vi "Configure Network De-embedding.vi"(0 "VISA resource name":refnum<visa-resource-name>, 1 "Channel (1)":i32=1, 2 "Network De-embeding State (F: Disable)":bool, 3 "Port 1 (1)":i32=1, 5 "Circuit Type (0: None)":u16(ring) items=["None", "User"], 11 "error in (no error)":errorcluster, 14 "File Name (\"\")":string) -> (4 "VISA resource name out":refnum<visa-resource-name>, 15 "error out":errorcluster)   [LabVIEW 2022 SP3, in "Agilent ENA Series.lvlib"]
doc: "Configures network de-embedding."
uses:
  <instrlib>/Agilent ENA Series/Agilent ENA Series.lvlib
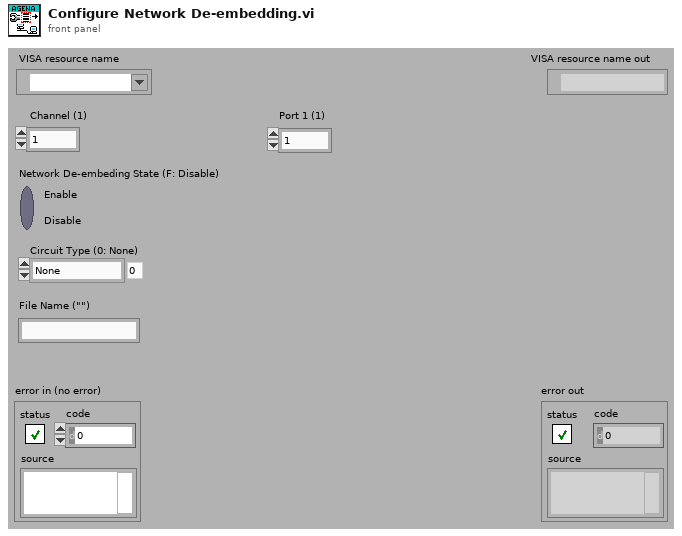
[diagram p1: front panel]
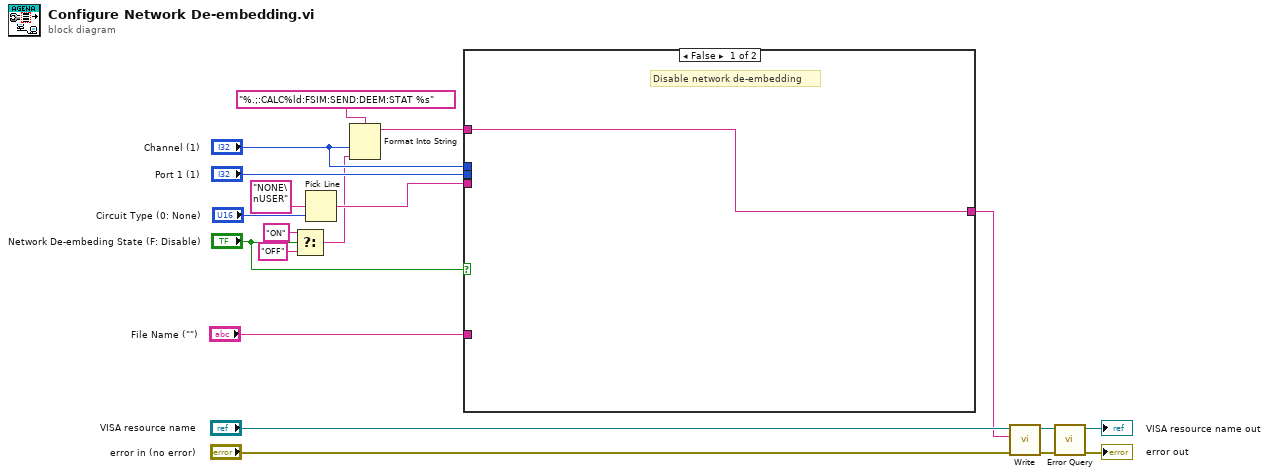
[diagram p0: block diagram]
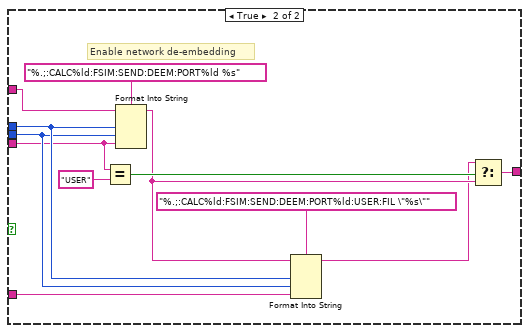
[diagram p2: hidden frame]
diagram:
  n1 = Select(t="ON", s="Network De-embeding State (F: Disable)", f="OFF") -> (s? t:f=w7:string)
  n2 = Pick Line(multi-line string="NONE\nUSER", line index="Circuit Type (0: None)") -> (output string=w12:string)  [unwired: 1 in]
  n3 = Format Into String(format string="%.;:CALC%ld:FSIM:SEND:DEEM:STAT %s", "Channel (1)", w7) -> (resulting string=w5:string)  [unwired: 2 in, 1 out]
  n4 = case shown="False" "Network De-embeding State (F: Disable)" {
    tunnel: "Channel (1)" -> [_ w28]
    tunnel: "Port 1 (1)" -> [_ w27]
    tunnel: w12 -> [_ w26]
    tunnel: "File Name (\"\")" -> [_ w21]
    tunnel: [w20 w23] -> w6
    tunnel: w5 -> [w20 w22]
    frame False {
      # "Disable network de-embedding"
    }
    frame True {
      # "Enable network de-embedding"
      n5 = Equal?(x=w26, y="USER") -> (x = y?=w30:bool)
      n6 = Format Into String(format string="%.;:CALC%ld:FSIM:SEND:DEEM:PORT%ld %s", initial string=w22, w28, w27, w26) -> (resulting string=w25:string)  [unwired: 1 in, 1 out]
      n7 = Format Into String(format string="%.;:CALC%ld:FSIM:SEND:DEEM:PORT%ld:USER:FIL \"%s\"" ("t"), initial string=w25, w28, w27, w21) -> (resulting string=w24:string)  [unwired: 1 in, 1 out]
      n8 = Select(t=w24, s=w30, f=w25) -> (s? t:f=w23:string)
    }
  }
  n9 = call <instrlib>:"Write.vi"("error in (no error)"="error in (no error)", "String ()"=w6, "VISA resource name"="VISA resource name") -> ("error out"=w3:errorcluster, "VISA resource name out"=w4:refnum<visa-resource-name>)  [unwired: 6 in, 1 out]
  n10 = call <instrlib>:"Error Query.vi"("error in (no error)"=w3, "VISA resource name"=w4) -> ("error out"=→"error out":errorcluster, "VISA resource name out"=→"VISA resource name out":refnum<visa-resource-name>)  [unwired: 6 in, 2 out]
